vi "CRIS requestor 2.vi"() -> ()   [LabVIEW 2013]
panel:
  out "PythonWaveReadback":dbl format="%.4f"
  out "PythonIsOK":bool
  out "Loop Counter":i32
  in  "Send Request":bool
  in  "WL request":dbl=10000.0 format="%.4f"
  in  "Stop Button":bool
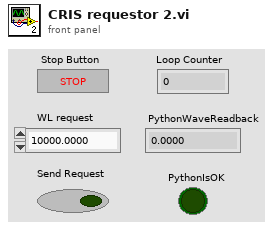
[diagram p1: front panel]
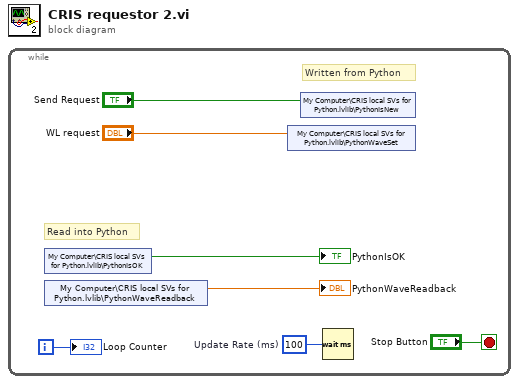
[diagram p0: block diagram]
diagram:
  n1 = while {
    i -> [w5]
    stop <- "Stop Button" stop-if-true
    w6 = u32 100  # Update Rate (ms)
    # "Read into Python"
    # "Written from Python"
    n2 = shared-variable "My Computer\\CRIS local SVs for Python.lvlib\\PythonIsOK"() -> (→"PythonIsOK":bool)  [unwired: 1 in, 1 out]
    n3 = shared-variable "My Computer\\CRIS local SVs for Python.lvlib\\PythonWaveReadback"() -> (→"PythonWaveReadback":dbl)  [unwired: 1 in, 1 out]
    n4 = shared-variable "My Computer\\CRIS local SVs for Python.lvlib\\PythonWaveSet"("WL request") -> ()  [unwired: 1 in, 1 out]
    n5 = shared-variable "My Computer\\CRIS local SVs for Python.lvlib\\PythonIsNew"("Send Request") -> ()  [unwired: 1 in, 1 out]
    n6 = Wait (ms)(milliseconds to wait=w6) -> ()  [unwired: 1 out]
    "Loop Counter" <- w5
  }
